vi "Build.vi"(7 "bulid type":T1, 8 "error in (no error)":errorcluster, 9 "save build info to solution":bool=TRUE, 11 "package builder solution path":path) -> (0 "error out":errorcluster, 3 "command line standard output":string)   [LabVIEW 2022 SP3, in "NI Package Builder API.lvlib"]
uses:
  NI Package Builder API.lvlib
  build type.ctl
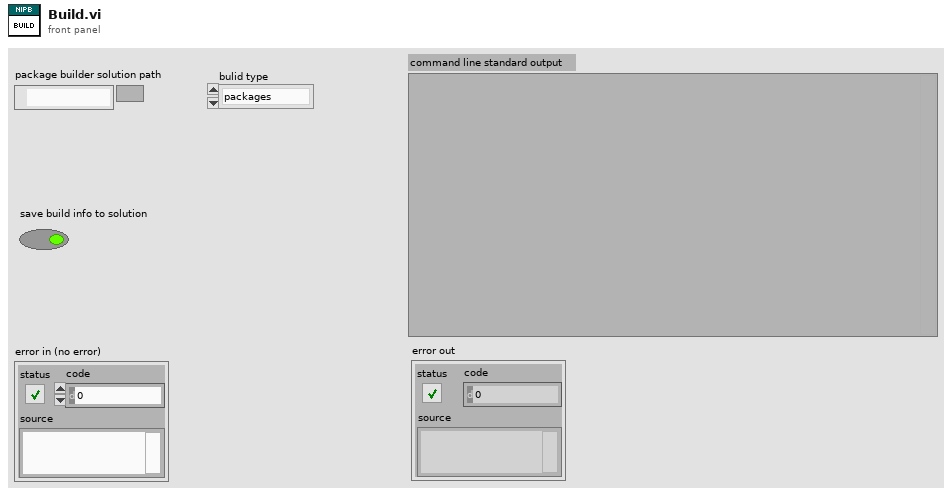
[diagram p1: front panel]
types:
  T1 = typedef "NI Package Builder API.lvlib/build type.ctl" = enum16{"packages", "feeds", "solution"}
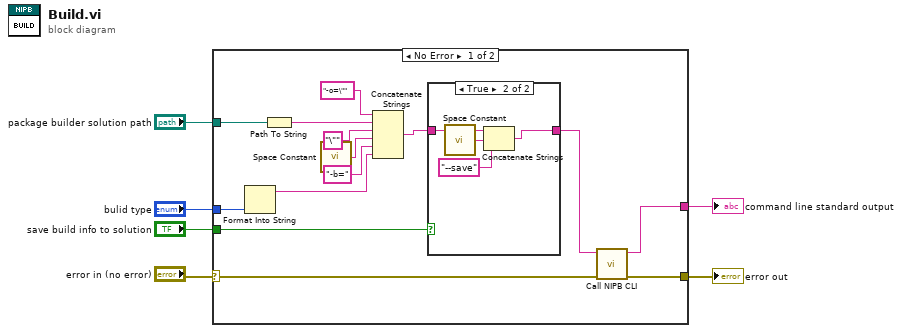
[diagram p0: block diagram]
diagram:
  n1 = case shown="No Error" "error in (no error)" {
    selector: "error in (no error)" -> [w7 w26]
    tunnel: [w20 w26] -> w6
    tunnel: "package builder solution path" -> [w18 _]
    tunnel: "bulid type" -> [w15 _]
    tunnel: "save build info to solution" -> [w12 _]
    tunnel: [w8 _] -> w2
    frame No Error {
      n2 = Format Into String(w15) -> (resulting string=w14:string)  [unwired: 3 in, 1 out]
      n3 = Path To String(path=w18) -> (string=w17:string)
      n4 = call <vilib>:"Space Constant.vi"() -> ("String"=w10:string)
      n5 = Concatenate Strings("-o=\"" ("string"), w17, "\"", w10, "-b=" ("string"), w14) -> (w13:string)
      n6 = case shown="True" w12 {
        tunnel: w13 -> [w21 w25]
        tunnel: [w21 w22] -> w11
        frame False {
        }
        frame True {
          n7 = call <vilib>:"Space Constant.vi"() -> ("String"=w24:string)
          n8 = Concatenate Strings(w25, w24, "--save" ("string")) -> (w22:string)
        }
      }
      n9 = call "Call NIPB CLI.vi"("error in (no error)"=w7, "command"=w11) -> ("error out"=w20:errorcluster, "command line standard output"=w8:string)  [unwired: 8 in]
    }
    frame Error {
    }
  }
  "error out" <- w6
  "command line standard output" <- w2
